vi "Pareto Random.vi"(6 "seed":i32=-1, 7 "reset":bool, 9 "c":dbl=3.0, 10 "a":dbl=1.0, 11 "samples":i32=128) -> (0 "error":i32, 3 "Pareto random data":dbl[](array[numeric])=[1.0200435724583867, 1.191186821381315, 1.3454787824274732, 3.2022994889318235, 3.298083870191973, 1.3440931502138358, 1.1536897087307796, 1.8358293081016885, 1.2315007579885913, 1.026998499181321, 1.132655859890926, 1.0506377476633444, 1.1400473541461857, 1.007271793010794, 1.379062009918852, 1.0603597382993417, 1.0419260337190315, 1.0826583583294245, 2.799090412068811, 1.8483191283561091, 2.1846956225092584, 1.3480524924666561, 1.9917009890447293, 1.2041965910871115, 1.7662198108427083, 1.4037653857572676, 1.2228758190929625, 1.0191360613583043, 1.0908616849657091, 4.550570845051509, 1.468881807879039, 3.1500520885498373, 1.174857802568457, 2.027359666592307, 1.361588361616142, 1.1994211617970763, 1.6860495709960965, 1.516324541504398, 1.9841983082686783, 1.9306923605003306, 1.0274002570803826, 1.3353856476190857, 1.2458141465905612, 1.418346149123217, 2.0575784186657695, 1.2083176424633117, 1.2943474924024791, 1.168660615384437, 1.2235182690187953, 1.7628539998376018, 1.0153532959260654, 1.3243449333011372, 1.0882880624464046, 1.597111415606967, 1.00628208742326, 1.0148048430102279, 1.042603500371912, 1.0760819902439833, 1.4542367257282032, 1.996934494065356, 1.4267389528130836, 1.1342167943697208, 1.1723166554149278, 1.1699657525914235, 1.1054162737676723, 1.2613371158530238, 1.0952237601229664, 1.053045064861921, 1.0716076074297627, 1.067611281547574, 1.257947679505888, 1.7405963904791388, 1.3280451283619905, 1.4613365967630794, 1.1817785594870318, 1.065665550326725, 1.5127085854789826, 1.8448385631018889, 1.1970864175058193, 1.004516108098263, 1.6958251741672892, 1.0429969810885544, 1.0041600540061084, 1.232650499316415, 1.1698189397138934, 1.0797762001825388, 1.177264524343754, 2.0971860681281314, 1.0970856904488393, 1.323220062003029, 1.0114286726555368, 1.020851934936706, 1.1705014122671231, 1.0358321552848169, 3.297056969589368, 2.070601460626365, 1.1799534830048575, 1.585352185662745, 1.116480411091954, 1.1827339480894783, 1.1694952015218028, 1.7601427413619268, 1.8260069679637607, 1.1260312686225347, 1.0211255891575677, 1.197389761769954, 1.1055373825248624, 1.3102557110090671, 1.0771056144484201, 1.9802518726469884, 1.1085061087352093, 1.0139671663864174, 1.1924147677215662, 2.125287759816924, 1.460770669873244, 1.1402792705177835, 1.170850109285882, 1.7928394347095038, 1.1166104444704685, 1.124726717859762, 1.05202223190346, 2.0960265025270104, 1.1920858159253875, 1.361287289907235, 1.1371582043363102, 1.1000149557182597, 1.028283452177441, 1.382493256907684])   [LabVIEW 2014, in "NI_Gmath.lvlib"]
doc: "Generates random values from a variate X, where X describes the selected distribution type. You must manually select the polymorphic instance to use."
uses:
  NI_Gmath.lvlib
  st_error_code.ctl
panel:
  # "Pareto Random"
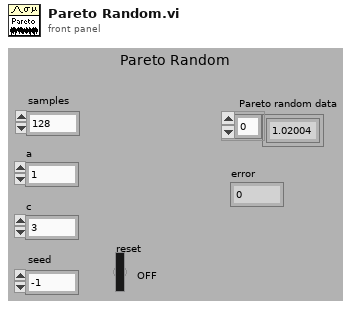
[diagram p1: front panel]
types:
  T1 = typedef "NI_Gmath.lvlib/st_error_code.ctl" = i32
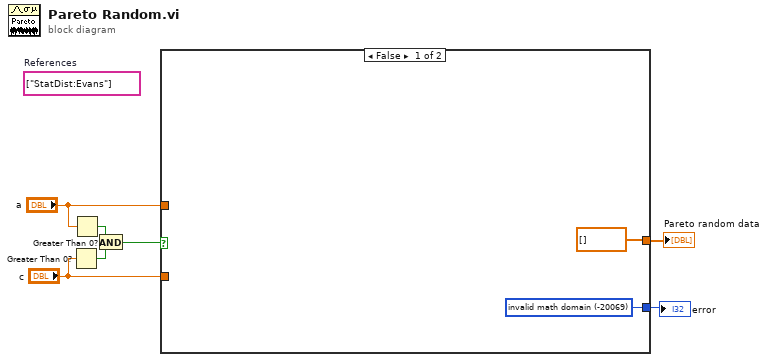
[diagram p0: block diagram]
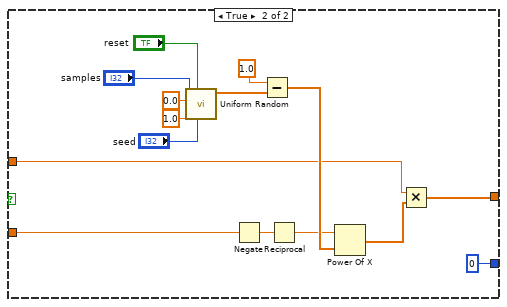
[diagram p2: hidden frame]
diagram:
  (unwired) string[] ["StatDist:Evans"]  # References
  n1 = Greater Than 0?(x="c") -> (x > 0?=w4:bool)
  n2 = Greater Than 0?(x="a") -> (x > 0?=w5:bool)
  n3 = And(x=w5, y=w4) -> (x .and. y?=w1:bool)
  n4 = case shown="False" w1 {
    tunnel: [w8 0 ("invalid math domain")] -> w7
    tunnel: [dbl[] [] w10] -> w6
    tunnel: "a" -> [_ w11]
    tunnel: "c" -> [_ w12]
    frame False {
      w8 = T1 -20069 items=["invalid math domain"=-20069, "Fourier interpolation size m >= n"=-20070, "empty array"=-20003] ("stat interp error code")
    }
    frame True {
      n5 = call "Uniform Random.vi"("seed"="seed", "reset"="reset", "xmax"=1.0, "xmin"=0.0, "samples"="samples") -> ("uniform random data"=w13:dbl[])  [unwired: 5 in, 1 out]
      n6 = Negate(x=w12) -> (-x=w15:dbl)
      n7 = Subtract(x=1.0, y=w13) -> (x-y=w16:dbl[])
      n8 = Reciprocal(x=w15) -> (1/x=w14:dbl)
      n9 = Power Of X(1:w16, 2:w14) -> (0:w17:dbl[])
      n10 = Multiply(x=w11, y=w17) -> (x*y=w10:dbl[])
    }
  }
  "error" <- w7
  "Pareto random data" <- w6
